vi "Double.to.BinaryShortPrice.vi"(11 "Double":dbl) -> (3 "BinaryLongPrice":u64 format="%.0x")   [LabVIEW 2020]
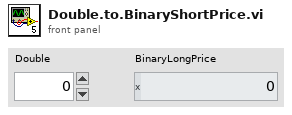
[diagram p1: front panel]
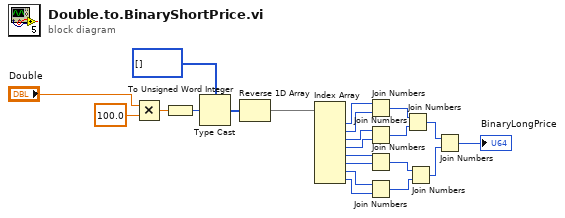
[diagram p0: block diagram]
diagram:
  n1 = Multiply(x="Double", y=100.0) -> (x*y=w4:dbl)
  n2 = To Unsigned Word Integer(number=w4) -> (unsigned 16bit integer=w3:u16)
  n3 = Type Cast(type=u8[] [], x=w3) -> (*(type *) &x=w2:u8[])
  n4 = Reverse 1D Array(array=w2) -> (reversed array=w20:u8[])
  n5 = Index Array(array=w20) -> (element #1=w22:u8, element #2=w7:u8, element #3=w8:u8, element #4=w9:u8, element #5=w10:u8, element #6=w11:u8, element #7=w12:u8, element #8=w13:u8)  [unwired: 8 in]
  n6 = Join Numbers(hi=w22, lo=w7) -> ((hi.lo)=w14:u16)
  n7 = Join Numbers(hi=w8, lo=w9) -> ((hi.lo)=w15:u16)
  n8 = Join Numbers(hi=w10, lo=w11) -> ((hi.lo)=w16:u16)
  n9 = Join Numbers(hi=w12, lo=w13) -> ((hi.lo)=w17:u16)
  n10 = Join Numbers(hi=w14, lo=w15) -> ((hi.lo)=w18:u32)
  n11 = Join Numbers(hi=w16, lo=w17) -> ((hi.lo)=w19:u32)
  n12 = Join Numbers(hi=w18, lo=w19) -> ((hi.lo)=→"BinaryLongPrice":u64)
